vi "LUT_Tetrominos.vi"() -> (0 "Init Data Out":fxp<+,6,6>[](array[numeric]))   [LabVIEW 2018]
panel:
  out "size(s)":i32
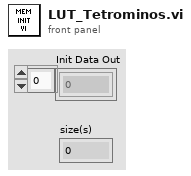
[diagram p1: front panel]
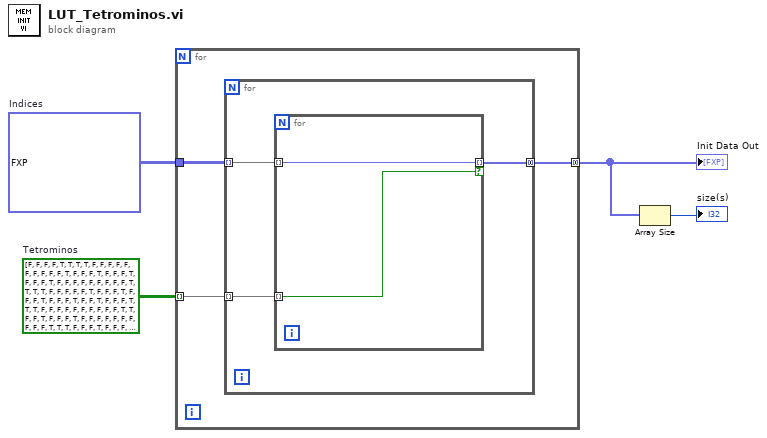
[diagram p0: block diagram]
diagram:
  w4 = bool[][][] [[[FALSE, FALSE, FALSE, FALSE], [TRUE, TRUE, TRUE, TRUE], [FALSE, FALSE, FALSE, FALSE], [FALSE, FALSE, FALSE, FALSE]], [[FALSE, FALSE, TRUE, FALSE], [FALSE, FALSE, TRUE, FALSE], [FALSE, FALSE, TRUE, FALSE], [FALSE, FALSE, TRUE, FALSE]], [[FALSE, FALSE, FALSE, FALSE], [FALSE, FALSE, FALSE, FALSE], [TRUE, TRUE, TRUE, TRUE], [FALSE, FALSE, FALSE, FALSE]], [[FALSE, TRUE, FALSE, FALSE], [FALSE, TRUE, FALSE, FALSE], [FALSE, TRUE, FALSE, FALSE], [FALSE, TRUE, FALSE, FALSE]], [[TRUE, FALSE, FALSE, FALSE], [TRUE, TRUE, TRUE, FALSE], [FALSE, FALSE, FALSE, FALSE], [FALSE, FALSE, FALSE, FALSE]], [[FALSE, TRUE, TRUE, FALSE], [FALSE, TRUE, FALSE, FALSE], [FALSE, TRUE, FALSE, FALSE], [FALSE, FALSE, FALSE, FALSE]], [[FALSE, FALSE, FALSE, FALSE], [TRUE, TRUE, TRUE, FALSE], [FALSE, FALSE, TRUE, FALSE], [FALSE, FALSE, FALSE, FALSE]], [[FALSE, TRUE, FALSE, FALSE], [FALSE, TRUE, FALSE, FALSE], [TRUE, TRUE, FALSE, FALSE], [FALSE, FALSE, FALSE, FALSE]], [[FALSE, FALSE, TRUE, FALSE], [TRUE, TRUE, TRUE, FALSE], [FALSE, FALSE, FALSE, FALSE], [FALSE, FALSE, FALSE, FALSE]], [[FALSE, TRUE, FALSE, FALSE], [FALSE, TRUE, FALSE, FALSE], [FALSE, TRUE, TRUE, FALSE], [FALSE, FALSE, FALSE, FALSE]], [[FALSE, FALSE, FALSE, FALSE], [TRUE, TRUE, TRUE, FALSE], [TRUE, FALSE, FALSE, FALSE], [FALSE, FALSE, FALSE, FALSE]], [[TRUE, TRUE, FALSE, FALSE], [FALSE, TRUE, FALSE, FALSE], [FALSE, TRUE, FALSE, FALSE], [FALSE, FALSE, FALSE, FALSE]], [[FALSE, TRUE, TRUE, FALSE], [FALSE, TRUE, TRUE, FALSE], [FALSE, FALSE, FALSE, FALSE], [FALSE, FALSE, FALSE, FALSE]], [[FALSE, TRUE, TRUE, FALSE], [FALSE, TRUE, TRUE, FALSE], [FALSE, FALSE, FALSE, FALSE], [FALSE, FALSE, FALSE, FALSE]], [[FALSE, TRUE, TRUE, FALSE], [FALSE, TRUE, TRUE, FALSE], [FALSE, FALSE, FALSE, FALSE], [FALSE, FALSE, FALSE, FALSE]], [[FALSE, TRUE, TRUE, FALSE], [FALSE, TRUE, TRUE, FALSE], [FALSE, FALSE, FALSE, FALSE], [FALSE, FALSE, FALSE, FALSE]], [[FALSE, TRUE, TRUE, FALSE], [TRUE, TRUE, FALSE, FALSE], [FALSE, FALSE, FALSE, FALSE], [FALSE, FALSE, FALSE, FALSE]], [[FALSE, TRUE, FALSE, FALSE], [FALSE, TRUE, TRUE, FALSE], [FALSE, FALSE, TRUE, FALSE], [FALSE, FALSE, FALSE, FALSE]], [[FALSE, FALSE, FALSE, FALSE], [FALSE, TRUE, TRUE, FALSE], [TRUE, TRUE, FALSE, FALSE], [FALSE, FALSE, FALSE, FALSE]], [[TRUE, FALSE, FALSE, FALSE], [TRUE, TRUE, FALSE, FALSE], [FALSE, TRUE, FALSE, FALSE], [FALSE, FALSE, FALSE, FALSE]], [[FALSE, TRUE, FALSE, FALSE], [TRUE, TRUE, TRUE, FALSE], [FALSE, FALSE, FALSE, FALSE], [FALSE, FALSE, FALSE, FALSE]], [[FALSE, TRUE, FALSE, FALSE], [FALSE, TRUE, TRUE, FALSE], [FALSE, TRUE, FALSE, FALSE], [FALSE, FALSE, FALSE, FALSE]], [[FALSE, FALSE, FALSE, FALSE], [TRUE, TRUE, TRUE, FALSE], [FALSE, TRUE, FALSE, FALSE], [FALSE, FALSE, FALSE, FALSE]], [[FALSE, TRUE, FALSE, FALSE], [TRUE, TRUE, FALSE, FALSE], [FALSE, TRUE, FALSE, FALSE], [FALSE, FALSE, FALSE, FALSE]], [[TRUE, TRUE, FALSE, FALSE], [FALSE, TRUE, TRUE, FALSE], [FALSE, FALSE, FALSE, FALSE], [FALSE, FALSE, FALSE, FALSE]], [[FALSE, FALSE, TRUE, FALSE], [FALSE, TRUE, TRUE, FALSE], [FALSE, TRUE, FALSE, FALSE], [FALSE, FALSE, FALSE, FALSE]], [[FALSE, FALSE, FALSE, FALSE], [TRUE, TRUE, FALSE, FALSE], [FALSE, TRUE, TRUE, FALSE], [FALSE, FALSE, FALSE, FALSE]], [[FALSE, TRUE, FALSE, FALSE], [TRUE, TRUE, FALSE, FALSE], [TRUE, FALSE, FALSE, FALSE], [FALSE, FALSE, FALSE, FALSE]]]  # Tetrominos
  w3 = fxp<+,6,6>[][] [[0.0, 1.0, 2.0, 3.0], [10.0, 11.0, 12.0, 13.0], [20.0, 21.0, 22.0, 23.0], [30.0, 31.0, 32.0, 33.0]]  # Indices
  n1 = for {
    tunnel: w4 -> [w7] mode=indexing
    tunnel: w3 -> [w6]
    tunnel: [w5] -> w2 mode=concatenating
    n2 = for {
      tunnel: w7 -> [w9] mode=indexing
      tunnel: w6 -> [w10] mode=indexing
      tunnel: [w8] -> w5 mode=concatenating
      n3 = for {
        tunnel: w10 -> [w12] mode=indexing
        tunnel: w9 -> [w11] mode=indexing
        tunnel: [w12] -> w8 mode=indexing if=w11
      }
    }
  }
  "Init Data Out" <- w2
  n4 = Array Size(array=w2) -> (size(s)=→"size(s)":i32)
